vi "TDT-Find Valid Device.vi"(7 "Acceptable Devices":T1[](array[typedef])=[enum."RX6", enum."RZ5", enum."RZ6"], 11 "error in (no error)":errorcluster) -> (4 "device":T2, 10 "Device":T1, 15 "error out":errorcluster)   [LabVIEW 2020]
uses:
  Typedefs/TDT-Output source.ctl
  Typedefs/TDT-Device ID.ctl
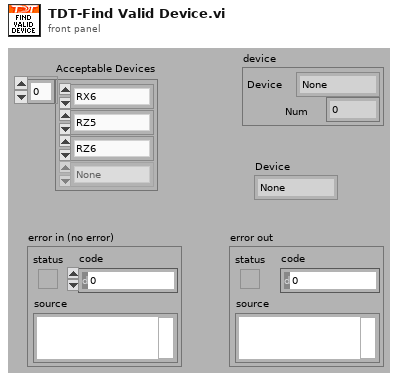
[diagram p1: front panel]
types:
  T1 = typedef "TDT-Device ID.ctl" = enum16{"None", "PA5", "RP2", "RL2", "RA16", "RV8", "RX5", "RX6", "RX7", "RX8", "RZ2", "RZ5", "RZ6"}
  T2 = typedef "TDT-Output source.ctl" = cluster{"Device":T1, "Num":i32}
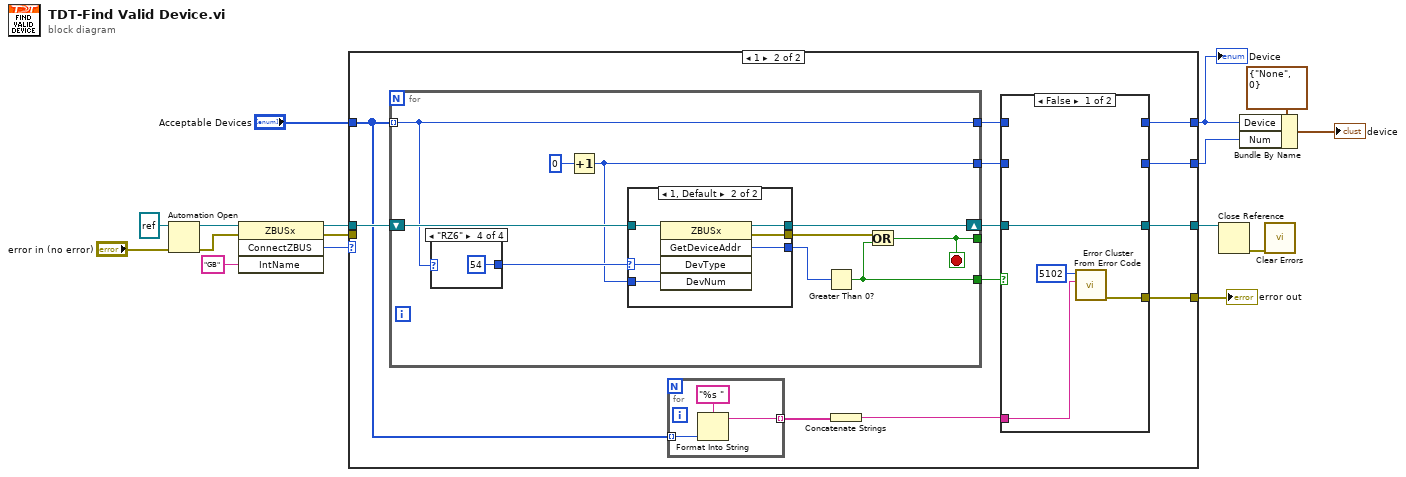
[diagram p0: block diagram]
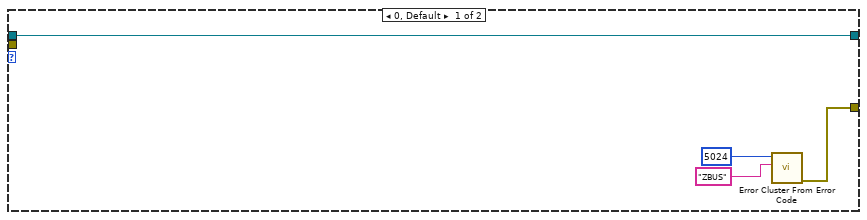
[diagram p2: hidden frame]
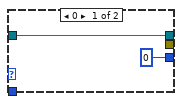
[diagram p4: hidden frame]
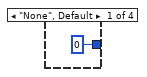
[diagram p5: hidden frame]
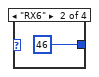
[diagram p6: hidden frame]
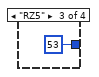
[diagram p7: hidden frame]
diagram:
  n1 = Automation Open(error in (no error)="error in (no error)", Automation Refnum=refnum<k7> refnum ("ZBUSXLib.ZBUSx")) -> (Automation Refnum=w11:refnum<k7>, error out=w12:errorcluster)  [unwired: 2 in]
  n2 = invoke class="ZBUSx" method="ConnectZBUS"(reference=w11, error in=w12, "IntName"="GB" ("ServerName")) -> (reference out=w8:refnum<k7>, error out=w14:errorcluster, "ConnectZBUS"=w13:i32)  [unwired: 1 in, 1 out]
  n3 = case shown="1" w13 {
    tunnel: w14 -> [_ _]
    tunnel: [w18 w26] -> w5
    tunnel: "Acceptable Devices" -> [_ w25]
    tunnel: w8 -> [w17 w32]
    tunnel: [_ w28] -> w2
    tunnel: [_ w27] -> w6
    tunnel: [w17 w21] -> w4
    frame 0, Default {
      n4 = call <vilib>:"Error Cluster From Error Code.vi"("error message (\"\")"="ZBUS" ("error message (\"\")"), "error code (0)"=5024) -> ("error out"=w18:errorcluster)  [unwired: 7 in]
    }
    frame 1 {
      n5 = for {
        tunnel: w25 -> [w49] mode=indexing
        tunnel: [w50] -> _
        tunnel: [w49] -> w29
        tunnel: [w48] -> w31
        tunnel: [w47] -> w30
        shift-right: [w46] -> w22
        shift-left: w32 -> [w52]
        stop <- w50 stop-if-true
        n6 = case shown="\"RZ6\"" w49 {
          tunnel: [0 ("DevType") 46 ("DevType") 53 ("DevType") 54 ("DevType")] -> w51
          frame "None", Default {
          }
          frame "RX6" {
          }
          frame "RZ5" {
          }
          frame "RZ6" {
          }
        }
        n7 = Increment(x=0) -> (x+1=w47:i32)
        n8 = case shown="1, Default" w51 {
          selector: w51 -> [_ w59]
          tunnel: w52 -> [w53 w60]
          tunnel: [_ w58] -> w44
          tunnel: w47 -> [_ w57]
          tunnel: [0 ("DevNum") w56] -> w45
          tunnel: [w53 w55] -> w46
          frame 0 {
          }
          frame 1, Default {
            n9 = invoke class="ZBUSx" method="GetDeviceAddr"(reference=w60, "DevType"=w59, "DevNum"=w57) -> (reference out=w55:refnum<k7>, error out=w58:errorcluster, "GetDeviceAddr"=w56:i32)  [unwired: 2 in, 2 out]
          }
        }
        n10 = Greater Than 0?(x=w45) -> (x > 0?=w48:bool)
        n11 = Or(x=w44, y=w48) -> (x .or. y?=w50:bool)
      }
      n12 = for {
        tunnel: w25 -> [w34] mode=indexing
        tunnel: [w33] -> w24 mode=indexing
        n13 = Format Into String(format string="%s ", w34) -> (resulting string=w33:string)  [unwired: 2 in, 1 out]
      }
      n14 = Concatenate Strings(w24) -> (w23:string)
      n15 = case shown="False" w31 {
        tunnel: w30 -> [_ w41]
        tunnel: w29 -> [_ w42]
        tunnel: [_ w42] -> w28
        tunnel: [_ w41] -> w27
        tunnel: [w38 _] -> w26
        tunnel: w23 -> [w37 _]
        tunnel: w22 -> [w36 w40]
        tunnel: [w36 w40] -> w21
        frame False {
          n16 = call <vilib>:"Error Cluster From Error Code.vi"("error message (\"\")"=w37, "error code (0)"=5102) -> ("error out"=w38:errorcluster)  [unwired: 7 in]
        }
        frame True {
        }
      }
    }
  }
  "error out" <- w5
  "Device" <- w2
  n17 = Close Reference(reference=w4) -> (error out=w3:errorcluster)  [unwired: 1 in]
  n18 = Bundle By Name(cluster=T2 {"Device"=enum."None", "Num"=0} ("device 2"), "Device"=w2, "Num"=w6) -> (→"device":T2)
  n19 = call <vilib>:"Clear Errors.vi"("error in (no error)"=w3) -> ()  [unwired: 5 in, 2 out]
